vi "Init Controls.vi"(8 "error in (no error)":errorcluster, 9 "SD Control Refs in":T2, 10 "SD Module in":refnum<class "SD Module.lvclass">, 11 "Node Ptr":T1 format="%.0x") -> (0 "error out":errorcluster, 1 "SD Control Refs out":T2, 2 "SD Module out":refnum<class "SD Module.lvclass">, 3 "Node Ptr":T1 format="%.0x", 5 "SubPanel Command":refnum<user-event>)   [LabVIEW 2019, in "Modules.lvlib" / "SD Module.lvclass"]
uses:
  SD Module.lvclass
  Type Defs/SD Control Refs.ctl
  Type Defs/Main Control Refs.ctl
  Type Defs/Counter Control Refs.ctl
  Type Defs/CDO Control Refs.ctl
  Type Defs/PWM Control Refs.ctl
  Type Defs/Quadrature Control Refs.ctl
  <vilib>/NI VeriStand/Custom Device API/Custom Device Item Ref.ctl
  RSI Module/SubPanel Command.ctl
  SD Module.lvclass/SD Module.ctl
  <vilib>/NI VeriStand/Custom Device API/Custom Device API.lvlib
  RSI Module/RSI Module.lvclass
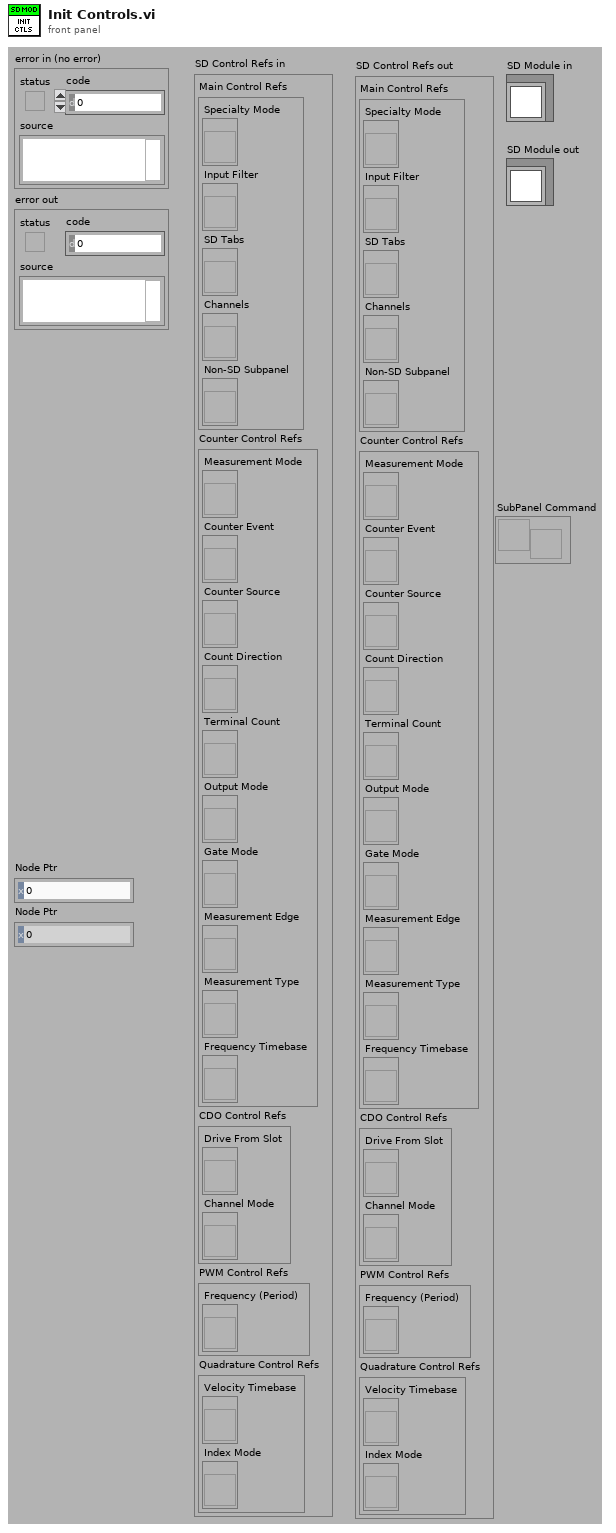
[diagram p1: front panel]
types:
  T1 = typedef "Custom Device API.lvlib/Custom Device Item Ref.ctl" = u64
  T2 = typedef "Modules.lvlib/SD Module.lvclass/SD Control Refs.ctl" = cluster{"Main Control Refs":T3, "Counter Control Refs":T4, "CDO Control Refs":T5, "PWM Control Refs":T6, "Quadrature Control Refs":T7}
  T3 = typedef "Modules.lvlib/SD Module.lvclass/Main Control Refs.ctl" = cluster{"Specialty Mode":refnum<vi>, "Input Filter":refnum<vi>, "SD Tabs":refnum<vi>, "Channels":refnum<vi>, "Non-SD Subpanel":refnum<vi>}
  T4 = typedef "Modules.lvlib/SD Module.lvclass/Counter Control Refs.ctl" = cluster{"Measurement Mode":refnum<vi>, "Counter Event":refnum<vi>, "Counter Source":refnum<vi>, "Count Direction":refnum<vi>, "Terminal Count":refnum<vi>, "Output Mode":refnum<vi>, "Gate Mode":refnum<vi>, "Measurement Edge":refnum<vi>, "Measurement Type":refnum<vi>, "Frequency Timebase":refnum<vi>}
  T5 = typedef "Modules.lvlib/SD Module.lvclass/CDO Control Refs.ctl" = cluster{"Drive From Slot":refnum<vi>, "Channel Mode":refnum<vi>}
  T6 = typedef "Modules.lvlib/SD Module.lvclass/PWM Control Refs.ctl" = cluster{"Frequency (Period)":refnum<vi>}
  T7 = typedef "Modules.lvlib/SD Module.lvclass/Quadrature Control Refs.ctl" = cluster{"Velocity Timebase":refnum<vi>, "Index Mode":refnum<vi>}
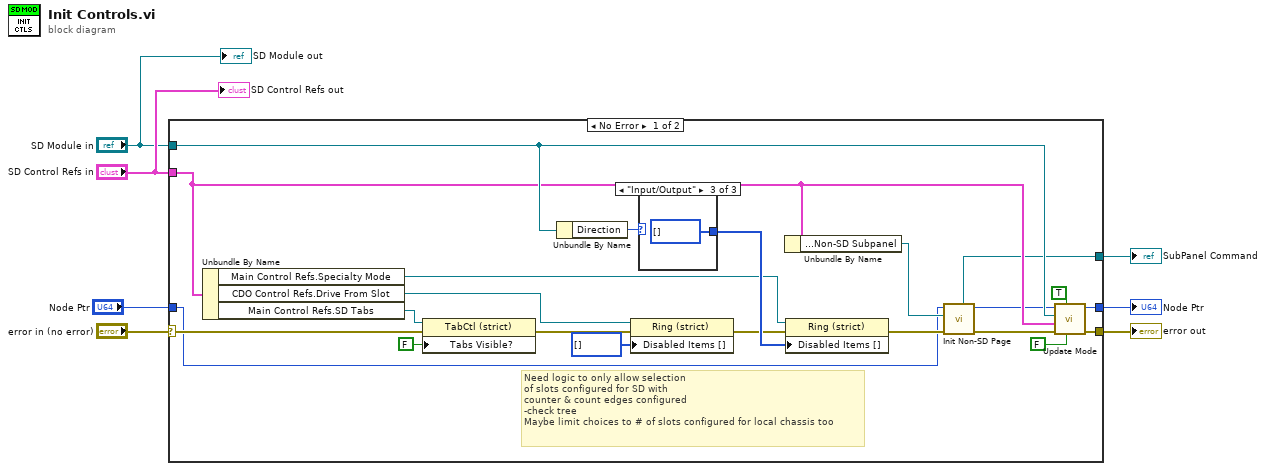
[diagram p0: block diagram]
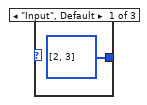
[diagram p2: hidden frame]
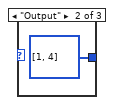
[diagram p3: hidden frame]
diagram:
  n1 = case shown="No Error" "error in (no error)" {
    selector: "error in (no error)" -> [w27 w34]
    tunnel: [w24 w34] -> w6
    tunnel: "SD Control Refs in" -> [w13 _]
    tunnel: "SD Module in" -> [w18 _]
    tunnel: "Node Ptr" -> [w11 w33]
    tunnel: [w17 w33] -> w2
    tunnel: [w9 _] -> w1
    frame No Error {
      # "Need logic to only allow selection\nof slots configured for SD with\ncounter & count edges configured\n-check tree\nMaybe limit choices to # of slots configured for local chassis too"
      n2 = Unbundle By Name(w13) -> ("Main Control Refs.Specialty Mode"=w23:refnum<vi>, "CDO Control Refs.Drive From Slot"=w21:refnum<vi>, "Main Control Refs.SD Tabs"=w29:refnum<vi>)
      n3 = property class="TabCtl (strict)"(reference=w29, error in=w27, "Tabs Visible?"=FALSE) -> (error out=w22:errorcluster)  [unwired: 1 out]
      n4 = Unbundle By Name(w18) -> ("Direction"=w26:enum16{"Input", "Output", "Input/Output"})
      n5 = property class="Ring (strict)"(reference=w21, error in=w22, "Disabled Items []"=i32[] []) -> (error out=w19:errorcluster)  [unwired: 1 out]
      n6 = case shown="\"Input/Output\"" w26 {
        tunnel: [i32[] [2, 3] ("Disabled Items []") i32[] [1, 4] ("Disabled Items []") i32[] [] ("Disabled Items []")] -> w25
        frame "Input", Default {
        }
        frame "Output" {
        }
        frame "Input/Output" {
        }
      }
      n7 = Unbundle By Name(w13) -> ("Main Control Refs.Non-SD Subpanel"=w12:refnum<vi>)
      n8 = property class="Ring (strict)"(reference=w23, error in=w19, "Disabled Items []"=w25) -> (error out=w15:errorcluster)  [unwired: 1 out]
      n9 = call "Init Non-SD Page.vi"("error in (no error)"=w15, "SubPanel Ref"=w12, "Node Ptr In"=w11) -> ("error out"=w14:errorcluster, "Node Ptr Out"=w10:T1, "SubPanel Command"=w9:refnum<user-event>)  [unwired: 5 in, 1 out]
      n10 = call "Update Mode.vi"("Refresh Channels? (T)"=FALSE, "Go to first chan?"=TRUE, "error in (no error)"=w14, "SD Control Refs in"=w13, "SD Module in"=w18, "Node Ptr In"=w10) -> ("error out"=w24:errorcluster, "Node Ptr Out"=w17:T1)  [unwired: 2 in, 2 out]
    }
    frame Error {
    }
  }
  "error out" <- w6
  "Node Ptr" <- w2
  "SubPanel Command" <- w1
  "SD Control Refs out" <- "SD Control Refs in"
  "SD Module out" <- "SD Module in"
